vi "Clear Panel Filter.vi"(8 "error in (no error)":errorcluster, 11 "2DArrayManager in":refnum<class "2DArrayManager.lvclass">) -> (0 "error out":errorcluster, 3 "2DArrayManager out":refnum<class "2DArrayManager.lvclass">)   [LabVIEW 2020, in "OOPanel.lvlib" / "2DArrayManager.lvclass"]
uses:
  2DArrayManager.lvclass
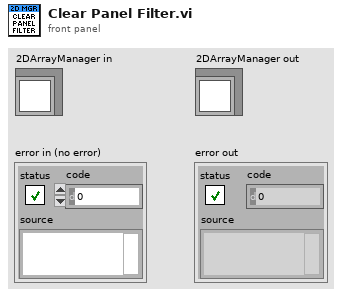
[diagram p1: front panel]
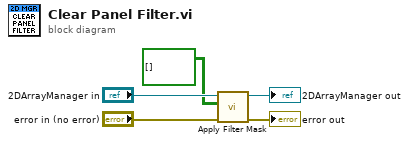
[diagram p0: block diagram]
diagram:
  n1 = call "Apply Filter Mask.vi"("error in (no error)"="error in (no error)", "Filter Mask"=bool[][] [], "2DArrayManager in"="2DArrayManager in") -> ("error out"=→"error out":errorcluster, "2DArrayManager out"=→"2DArrayManager out":refnum<class "2DArrayManager.lvclass">)  [unwired: 7 in]
